vi "String to Data Type.vi"(8 "error in (no error)":errorcluster, 11 "Date Type String":string) -> (0 "error out":errorcluster, 3 "Data Type":T1(ring)=enum."double")   [LabVIEW 2024]
doc: "Converts a string to a data type and generates a user-defined error if the conversion fails."
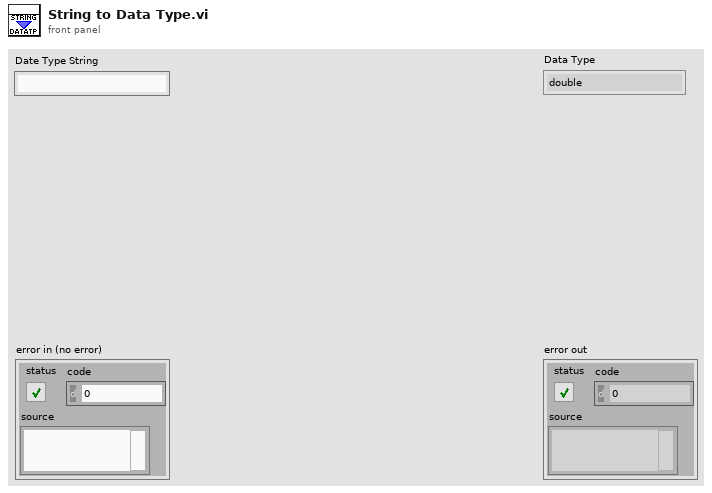
[diagram p1: front panel]
types:
  T1 = enum32{"u32BitField", "bool", "double", "string", "int8", "uint8", "int16", "uint16", "int32", "uint32", "int64", "uint64", "single", "double waveform", "int16 waveform", "array of boolean", "array of int8", "array of uint8", "array of int16", "array of uint16", "array of int32", "array of uint32", "array of int64", "array of uint64", "array of single", "array of double", "array of double waveform", "array of int16 waveform", "array of string", "variant", "timestamp", "fixed point", "custom"}
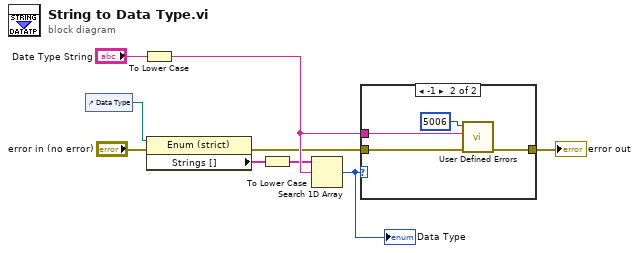
[diagram p0: block diagram]
diagram:
  n1 = control-ref of="Data Type"() -> (w9:refnum<vi>)
  n2 = To Lower Case(string="Date Type String") -> (all lower case string=w7:string)
  n3 = property on="Property Node" class="Enum (strict)"(reference=w9, error in="error in (no error)") -> (error out=w1:errorcluster, "Strings []"=w5:string[])  [unwired: 1 out]
  n4 = To Lower Case(string=w5) -> (all lower case string=w4:string[])
  n5 = Search 1D Array(1D array=w4, element=w7) -> (index of element=w3:i32)  [unwired: 1 in]
  "Data Type" <- w3
  n6 = case shown="-1" w3 {
    tunnel: w7 -> [_ w12]
    tunnel: [w10 w13] -> w6
    tunnel: w1 -> [w10 w11]
    frame Default {
    }
    frame -1 {
      n7 = call "User Defined Errors.vi"("error in (no error)"=w11, "Parameter 1"=w12, "Error Code (0)"=5006 ("error code (0)")) -> ("error out"=w13:errorcluster)  [unwired: 8 in]
    }
  }
  "error out" <- w6
